vi "1_2_front.vi"(11 "Formatted 1D String Array":string[](array[string])) -> (3 "Array":string[](array[string]))   [LabVIEW 2021, in "2023.lvlib"]
uses:
  2023.lvlib
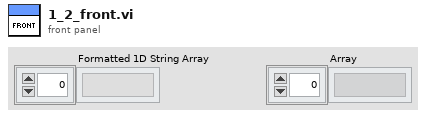
[diagram p1: front panel]
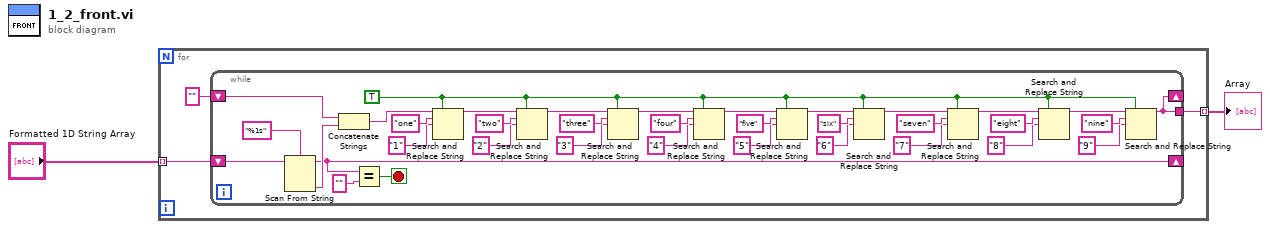
[diagram p0: block diagram]
diagram:
  n1 = for {
    tunnel: "Formatted 1D String Array" -> [w4] mode=indexing
    tunnel: [w5] -> w1 mode=indexing
    n2 = while {
      tunnel: [w6] -> w5
      shift-right: [w9] -> _
      shift-left: w4 -> [w14]
      shift-right: [w6] -> _
      shift-left: "" -> [w11]
      stop <- w7 stop-if-true
      w17 = TRUE ("replace all? (F)")
      n3 = Scan From String(format string="%1s", input string=w14) -> (remaining string=w9:string, output 1=w12:string)  [unwired: 3 in, 2 out]
      n4 = Concatenate Strings(w11, w12) -> (w10:string)
      n5 = Equal?(x=w9, y="") -> (x = y?=w7:bool)
      n6 = Search and Replace String(replace all?=w17, input string=w10, search string="one", replace string="1" ("replace string (\"\")")) -> (result string=w39:string)  [unwired: 4 in, 3 out]
      n7 = Search and Replace String(replace all?=w17, input string=w39, search string="two", replace string="2" ("replace string (\"\")")) -> (result string=w36:string)  [unwired: 4 in, 3 out]
      n8 = Search and Replace String(replace all?=w17, input string=w36, search string="three", replace string="3" ("replace string (\"\")")) -> (result string=w35:string)  [unwired: 4 in, 3 out]
      n9 = Search and Replace String(replace all?=w17, input string=w35, search string="four", replace string="4" ("replace string (\"\")")) -> (result string=w34:string)  [unwired: 4 in, 3 out]
      n10 = Search and Replace String(replace all?=w17, input string=w34, search string="five", replace string="5" ("replace string (\"\")")) -> (result string=w33:string)  [unwired: 4 in, 3 out]
      n11 = Search and Replace String(replace all?=w17, input string=w33, search string="six", replace string="6" ("replace string (\"\")")) -> (result string=w32:string)  [unwired: 4 in, 3 out]
      n12 = Search and Replace String(replace all?=w17, input string=w32, search string="seven", replace string="7" ("replace string (\"\")")) -> (result string=w21:string)  [unwired: 4 in, 3 out]
      n13 = Search and Replace String(replace all?=w17, input string=w21, search string="eight", replace string="8" ("replace string (\"\")")) -> (result string=w18:string)  [unwired: 4 in, 3 out]
      n14 = Search and Replace String(replace all?=w17, input string=w18, search string="nine", replace string="9" ("replace string (\"\")")) -> (result string=w6:string)  [unwired: 4 in, 3 out]
    }
  }
  "Array" <- w1
